vi "Solartron 1260 singlefile freq scan feb 15.vi"() -> ()   [LabVIEW 2014]
doc: "This VI configures and reads back a single measurement. \n\nNote:\nYou might need to extend the timeout set in the Wait Conditions subVI."
uses:
  <vilib>/Utility/file.llb/Write To Spreadsheet File (string).vi
  <instrlib>/Solartron 1260/Solartron 1260.lvlib
panel:
  in  "stop 2":bool
  out "File path":path
  out "XY Graph 4":cluster{dbl[], dbl[]}[](graph)
  in  "Variable, result source, citcuit 2":T1={"Variable (0:Frequency)"=enum."Frequency", "Result Source(0:Z1 = V1/I)"=enum."Z1 = V1/I", "Circuit (3:Parallel C, R)"=enum."Serial L, R", "Result Type(0: [Z, Theta] for: Z1 or Z2)"=enum."[Z, Theta]       for: Z1 or Z2", "DC Bias (V)"=0.0, "Amplitude (V)"=1.0} {"Amplitude (V)" min=0.0 max=3.0 format="%^.3e"; "DC Bias (V)" min=-42.0 max=42.0 format="%^.3e"}
  in  "measure spectrum":bool
  out "Scan time (hrs)":dbl
  out "Scan time (min)":dbl
  in  "stop":bool
  out "Freq. resolution (Hz)":dbl
  in  "Frequency options":T2={"End freq (Hz)"=0.0, "Start freq (Hz)"=0.0, "# of steps"=0.0, "# of steps to average"=3.0} {"Start freq (Hz)" format="%#_8f"; "End freq (Hz)" format="%#_8f"}
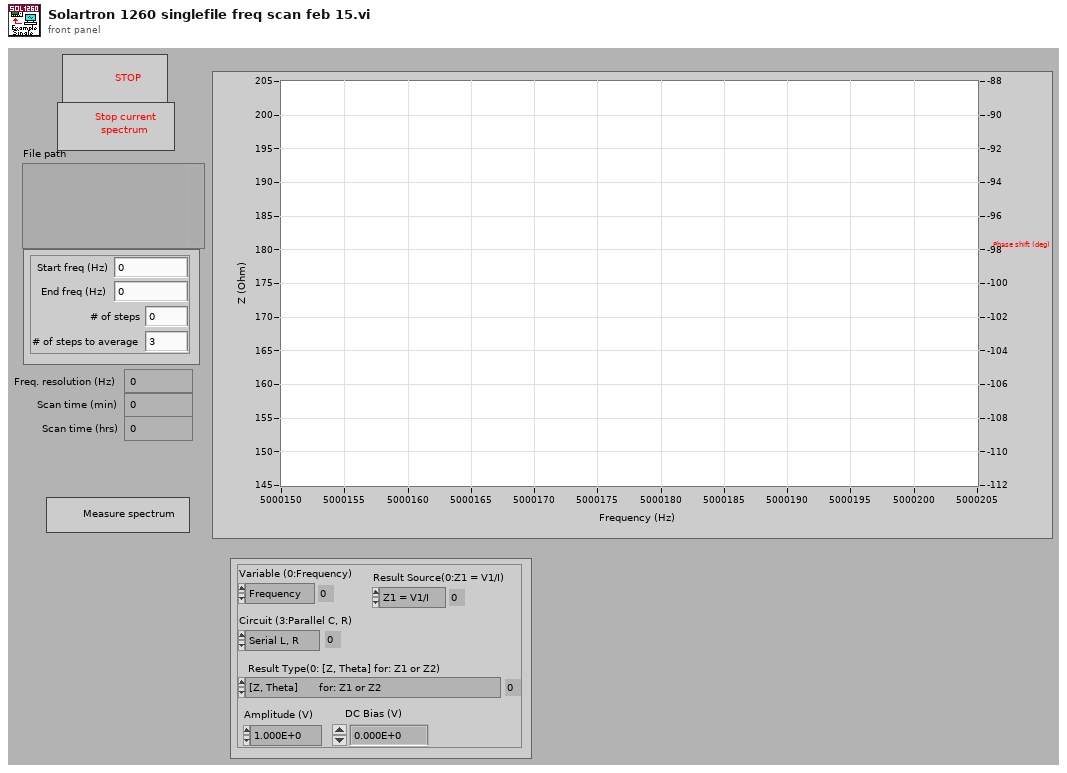
[diagram p1: front panel]
types:
  T1 = cluster{"Variable (0:Frequency)":enum16{"Frequency", "Amplitude", "Baise"}, "Result Source(0:Z1 = V1/I)":enum16{"Z1 = V1/I", "Y1 = I/V1", "Z2 = V2/I", "Y2 = I/V2", "Function (  )", "V1", "V2", "V1/V2", "V2/V1", " I"}, "Circuit (3:Parallel C, R)":enum16{"Serial L, R", "Serial C, R", "Parallel L, R", "Parallel C, R", "Auto"}, "Result Type(0: [Z, Theta] for: Z1 or Z2)":enum16{"[Z, Theta]       for: Z1 or Z2", "[Y, Theta]       for: Y1 or Y2", "[r, Theta]        for: Fnc( ), V1, V2, V1/V2, V2/V1 or I", "[r(dB), Theta]  for: Fnc( ), V1, V2, V1/V2 or V2/V1", "[r, t]                 for: Fnc( ), V1, V2, V1/V2 or V2/V1", "[r (dB), t]          for: Fnc( ), V1, V2, V1/V2 or V2/V1", "[L(or C), R]      for: Z1, Y1, Z2, Y2 or Fnc( )", "[L(or C), Q]      for: Z1, Y1, Z2, Y2 or Fnc( )", "[L(or C), D]      for: Z1, Y1, Z2, Y2 or Fnc( ) ", "[R, X]              for: Z1 or Z2", "[G, B]              for: Y1 or Y2", "[a, b]               for: Fnc( ), V1, V2, V1/V2, V2/V1 or I"}, "DC Bias (V)":dbl, "Amplitude (V)":dbl}
  T2 = cluster{"End freq (Hz)":dbl, "Start freq (Hz)":dbl, "# of steps":dbl, "# of steps to average":dbl}
  T3 = enum16{"Off", "All", "Fail", "Pass", "Dump", "Dump all", "Plotter"}
  T4 = enum16{"Z1 = V1/I", "Y1 = I/V1", "Z2 = V2/I", "Y2 = I/V2", "Function (  )", "V1", "V2", "V1/V2", "V2/V1", " I"}
  T5 = enum16{"Serial L, R", "Serial C, R", "Parallel L, R", "Parallel C, R", "Auto"}
  T6 = enum16{"[Z, Theta]       for: Z1 or Z2", "[Y, Theta]       for: Y1 or Y2", "[r, Theta]        for: Fnc( ), V1, V2, V1/V2, V2/V1 or I", "[r(dB), Theta]  for: Fnc( ), V1, V2, V1/V2 or V2/V1", "[r, t]                 for: Fnc( ), V1, V2, V1/V2 or V2/V1", "[r (dB), t]          for: Fnc( ), V1, V2, V1/V2 or V2/V1", "[L(or C), R]      for: Z1, Y1, Z2, Y2 or Fnc( )", "[L(or C), Q]      for: Z1, Y1, Z2, Y2 or Fnc( )", "[L(or C), D]      for: Z1, Y1, Z2, Y2 or Fnc( ) ", "[R, X]              for: Z1 or Z2", "[G, B]              for: Y1 or Y2", "[a, b]               for: Fnc( ), V1, V2, V1/V2, V2/V1 or I"}
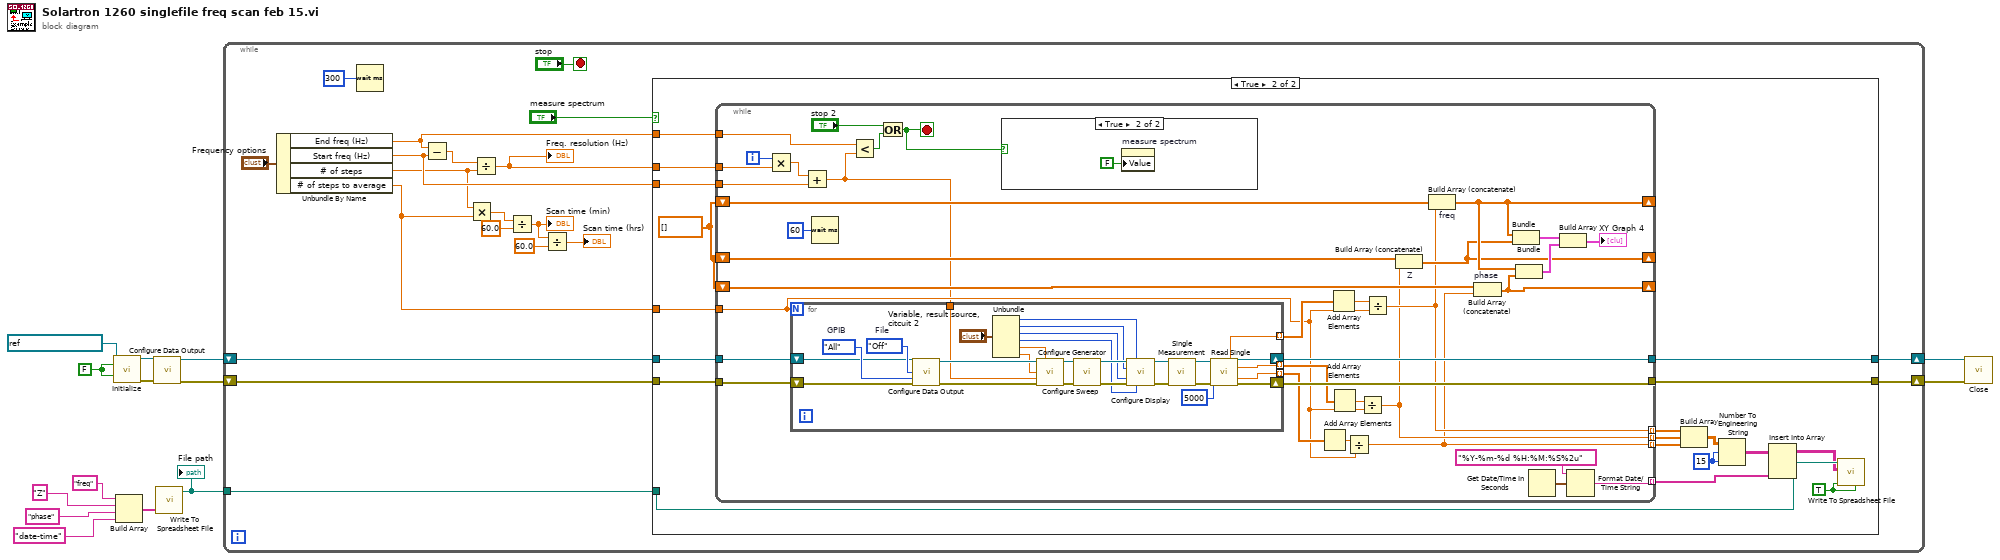
[diagram p0: block diagram]
diagram:
  w12 = FALSE ("ID Query (T: Check)")
  n1 = call <instrlib>:"Initialize.vi"("VISA resource name"=refnum<visa-resource-name> "GPIB2::4::INSTR", "ID Query (T: Check)"=w12, "Reset (T: Reset)"=w12) -> ("VISA resource name out"=w9:refnum<visa-resource-name>, "error out"=w10:errorcluster)  [unwired: 11 in]
  n2 = Build Array("freq", "Z", "phase", "date-time") -> (w3:string[])
  n3 = call <instrlib>:"Configure Data Output.vi"("VISA resource name"=w9, "error in (no error)"=w10) -> ("VISA resource name out"=w8:refnum<visa-resource-name>, "error out"=w7:errorcluster)  [unwired: 12 in]
  n4 = call-poly <vilib>:"Write To Spreadsheet File.vi"("1D data"=w3) -> ("new file path (Not A Path if cancelled)"=w2:path)  [unwired: 7 in]
  "File path" <- w2
  n5 = while {
    shift-right: [w32] -> w13
    shift-left: w8 -> [w31]
    shift-right: [w33] -> w14
    shift-left: w7 -> [w30]
    tunnel: w2 -> [w15]
    stop <- "stop" stop-if-true
    n6 = Unbundle By Name("Frequency options") -> ("End freq (Hz)"=w27:dbl, "Start freq (Hz)"=w28:dbl, "# of steps"=w22:dbl, "# of steps to average"=w20:dbl)
    n7 = Wait (ms)(milliseconds to wait=300) -> ()  [unwired: 1 out]
    n8 = Subtract(x=w27, y=w28) -> (x-y=w34:dbl)
    n9 = Multiply(x=w22, y=w20) -> (x*y=w21:dbl)
    n10 = Divide(x=w34, y=w22) -> (x/y=w19:dbl)
    "Freq. resolution (Hz)" <- w19
    n11 = Divide(x=w21, y=60.0) -> (x/y=w24:dbl)
    "Scan time (min)" <- w24
    n12 = Divide(x=w24, y=60.0) -> (x/y=→"Scan time (hrs)":dbl)
    n13 = case shown="True" "measure spectrum" {
      tunnel: [w35 w55] -> w33
      tunnel: [w36 w54] -> w32
      tunnel: w31 -> [w36 w53]
      tunnel: w30 -> [w35 w52]
      tunnel: w28 -> [_ w51]
      tunnel: w27 -> [_ w50]
      tunnel: w20 -> [_ w49]
      tunnel: w19 -> [_ w48]
      tunnel: w15 -> [_ w44]
      frame False {
      }
      frame True {
        w45 = TRUE ("append to file? (new file:F)")
        w46 = i16 15 ("precision (6)")
        w47 = dbl[] []
        n14 = while {
          tunnel: [w85] -> w55
          tunnel: [w84] -> w54
          tunnel: w53 -> [w87]
          tunnel: w52 -> [w86]
          tunnel: w51 -> [w88]
          shift-right: [w75] -> _
          shift-left: w47 -> [w83]
          shift-right: [w74] -> _
          shift-left: w47 -> [w82]
          tunnel: w48 -> [w81]
          shift-right: [w77] -> _
          shift-left: w47 -> [w78]
          tunnel: [w69] -> w43 mode=indexing
          tunnel: [w65] -> w41 mode=indexing
          tunnel: [w64] -> w42 mode=indexing
          tunnel: w50 -> [w63]
          tunnel: w49 -> [w68]
          tunnel: [w56] -> w39 mode=indexing
          i -> [w90]
          stop <- w59 stop-if-true
          n15 = Multiply(x=w90, y=w81) -> (x*y=w89:dbl)
          n16 = Add(x=w89, y=w88) -> (x+y=w62:dbl)
          n17 = for {
            N: w68 -> [_]
            tunnel: [w98] -> w73 mode=indexing
            tunnel: [w97] -> w72 mode=indexing
            tunnel: [w96] -> w71 mode=indexing
            tunnel: w62 -> [w95]
            shift-right: [w104] -> w84
            shift-left: w87 -> [w107]
            shift-right: [w105] -> w85
            shift-left: w86 -> [w106]
            w109 = T3."All"  # GPIB
            w110 = enum16{"Off", "All", "Fail", "Pass"}."Off"  # File
            n18 = call <instrlib>:"Configure Data Output.vi"("VISA resource name"=w107, "File (1:All)"=w110, "GPIB (1:All)"=w109, "error in (no error)"=w106) -> ("VISA resource name out"=w119:refnum<visa-resource-name>, "error out"=w120:errorcluster)  [unwired: 10 in]
            n19 = Unbundle("Variable, result source, citcuit 2") -> ("Variable (0:Frequency)"=w102:enum16{"Frequency", "Amplitude", "Baise"}, "Result Source(0:Z1 = V1/I)"=w100:T4, "Circuit (3:Parallel C, R)"=w101:T5, "Result Type(0: [Z, Theta] for: Z1 or Z2)"=w99:T6, "DC Bias (V)"=w94:dbl, "Amplitude (V)"=w93:dbl)
            n20 = call <instrlib>:"Configure Generator.vi"("VISA resource name"=w119, "Voltage Bias(0.0 V)"=w94, "Voltage Amplitude(1.0 V)"=w93, "Frequency(1.0 Hz)"=w95, "error in (no error)"=w120) -> ("VISA resource name out"=w118:refnum<visa-resource-name>, "error out"=w117:errorcluster)  [unwired: 9 in]
            n21 = call <instrlib>:"Configure Sweep.vi"("VISA resource name"=w118, "error in (no error)"=w117) -> ("VISA resource name out"=w115:refnum<visa-resource-name>, "error out"=w116:errorcluster)  [unwired: 12 in]
            n22 = call <instrlib>:"Configure Display.vi"("VISA resource name"=w115, "Variable (0:Frequency)"=w102, "Result Source(0:Z1 = V1/I)"=w100, "Circuit (3:Parallel C, R)"=w101, "error in (no error)"=w116, "Result Type(0: [Z, Theta] for: Z1 or Z2)"=w99) -> ("VISA resource name out"=w114:refnum<visa-resource-name>, "error out"=w113:errorcluster)  [unwired: 8 in]
            n23 = call <instrlib>:"Single Measurement.vi"("VISA resource name"=w114, "error in (no error)"=w113) -> ("VISA resource name out"=w111:refnum<visa-resource-name>, "error out"=w112:errorcluster)  [unwired: 12 in]
            n24 = call <instrlib>:"Read Single.vi"("VISA resource name"=w111, "timeout ms (5000)"=u32 5000, "error in (no error)"=w112) -> ("Variable"=w98:dbl, "VISA resource name out"=w104:refnum<visa-resource-name>, "Parameter 1"=w97:dbl, "Parameter2"=w96:dbl, "error out"=w105:errorcluster)  [unwired: 6 in, 2 out]
          }
          n25 = Wait (ms)(milliseconds to wait=u32 60) -> ()  [unwired: 1 out]
          n26 = Less?(x=w63, y=w62) -> (x < y?=w61:bool)
          n27 = Or(x="stop 2", y=w61) -> (x .or. y?=w59:bool)
          n28 = case shown="True" w59 {
            frame False {
            }
            frame True {
              n29 = property on="measure spectrum" class="Bool (strict)"("Value"=FALSE ("measure spectrum")) -> ()  [unwired: 2 in, 2 out]
            }
          }
          n30 = Add Array Elements(numeric array=w71) -> (sum=w67:dbl)
          n31 = Add Array Elements(numeric array=w73) -> (sum=w70:dbl)
          n32 = Add Array Elements(numeric array=w72) -> (sum=w66:dbl)
          n33 = Divide(x=w67, y=w68) -> (x/y=w64:dbl)
          n34 = Divide(x=w66, y=w68) -> (x/y=w65:dbl)
          n35 = Divide(x=w70, y=w68) -> (x/y=w69:dbl)
          n36 = Build Array (concatenate) "Z"(w82, w65) -> (w74:dbl[])
          n37 = Build Array (concatenate) "freq"(w83, w69) -> (w75:dbl[])
          n38 = Build Array (concatenate) "phase"(w78, w64) -> (w77:dbl[])
          n39 = Bundle(w75, w74) -> (w80:cluster{dbl[], dbl[]})  [unwired: 1 in]
          n40 = Bundle(w75, w77) -> (w79:cluster{dbl[], dbl[]})  [unwired: 1 in]
          n41 = Get Date/Time In Seconds() -> (seconds since 1Jan1904=w58:timestamp)
          n42 = Build Array(w80, w79) -> (→"XY Graph 4":cluster{dbl[], dbl[]}[])
          n43 = Format Date/Time String(time format string (%c)="%Y-%m-%d %H:%M:%S%2u", seconds (now)=w58) -> (date/time string=w56:string)  [unwired: 1 in]
        }
        n44 = Build Array(w43, w41, w42) -> (w38:dbl[][])
        n45 = Number To Engineering String(2:w46, 3:w46, 4:w38) -> (0:w40:string[][])  [unwired: 1 in]
        n46 = Insert Into Array(array=w40, new element=w39) -> (w37:string[][])  [unwired: 2 in]
        n47 = call-poly <vilib>:"Write To Spreadsheet File.vi"("transpose? (no:F)"=w45, "append to file? (new file:F)"=w45, "2D data"=w37, "file path (dialog if empty)"=w44) -> ()  [unwired: 4 in, 1 out]
      }
    }
  }
  n48 = call <instrlib>:"Close.vi"("VISA resource name"=w13, "error in (no error)"=w14) -> ()  [unwired: 13 in, 1 out]
